vi "NumIntegrate_Rkf45_Func_B2.vi"(11 "Index":i32) -> (3 "RKF45_B2":dbl)   [LabVIEW 2019, in "Trajectory_Library.lvlib"]
doc: "Internal function used by Rkdp_Impl.vi\n\nInputs:\n - Index -- Index into B2 array (must be 0 - 6 )\n\nOutputs:\n - B2 -- Value looked up by index."
uses:
  Trajectory_Library.lvlib
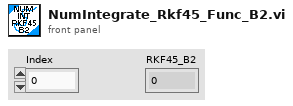
[diagram p1: front panel]
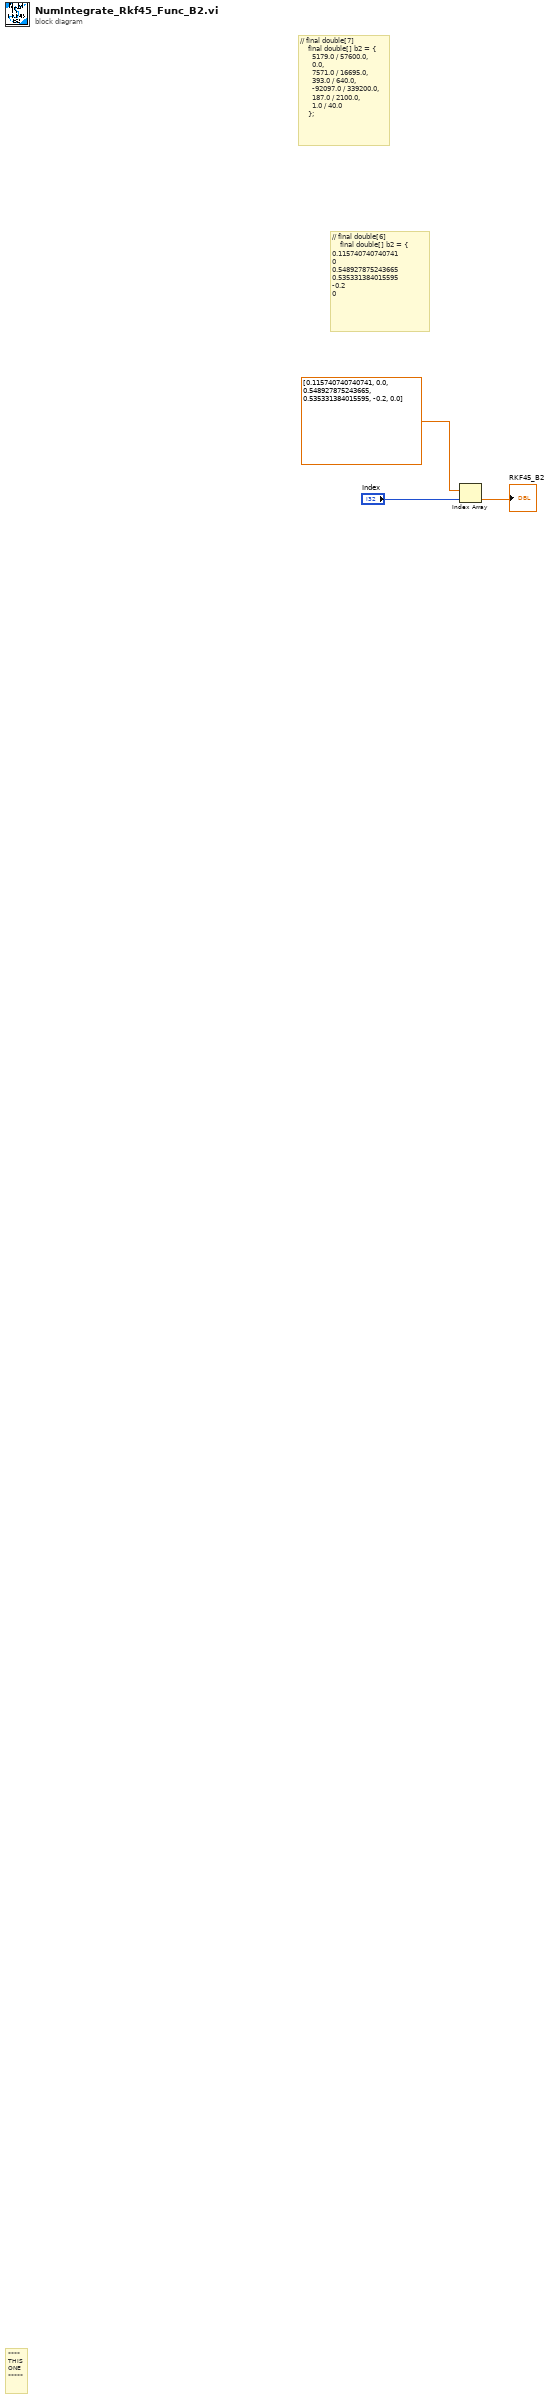
[diagram p0: block diagram]
diagram:
  # "// final double[6]\t\t\t\t\t\n    final double[] b2 = {\t\t\t\t\t\n0.115740740740741\t\n0\t\n0.548927875243665\t\n0.535331384015595\t\n-0.2\t\n0"
  # "// final double[7]\n    final double[] b2 = {\n      5179.0 / 57600.0,\n      0.0,\n      7571.0 / 16695.0,\n      393.0 / 640.0,\n      -92097.0 / 339200.0,\n      187.0 / 2100.0,\n      1.0 / 40.0\n    };"
  # "****\nTHIS\nONE\n*****"
  n1 = Index Array(array=dbl[] [0.115740740740741, 0.0, 0.548927875243665, 0.535331384015595, -0.2, 0.0], index="Index") -> (element=→"RKF45_B2":dbl)
